vi "String_Parsing.vi"(7 "Search_Params":string[](array[string])=["x1", "y1", "z1", "x2", "y2", "z2"], 11 "Input":string) -> (3 "Positions":i32[](array[numeric]))   [LabVIEW 2016]
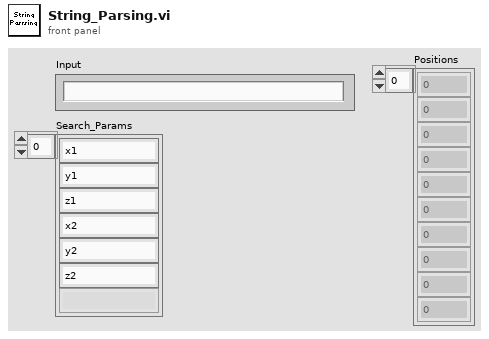
[diagram p1: front panel]
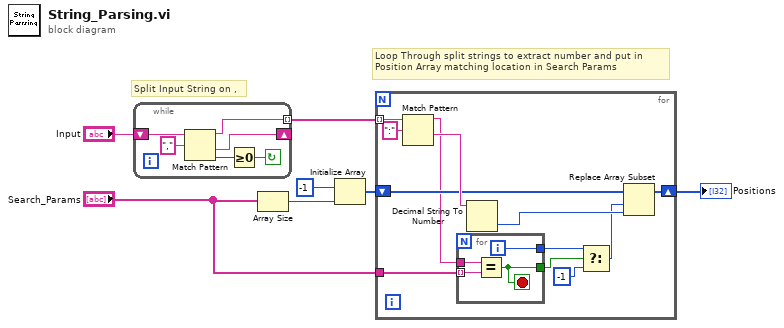
[diagram p0: block diagram]
diagram:
  # "Loop Through split strings to extract number and put in\nPosition Array matching location in Search Params"
  # "Split Input String on ,"
  n1 = while {
    shift-right: [w10] -> _
    shift-left: "Input" -> [w13]
    tunnel: [w11] -> w6 mode=indexing
    stop <- w8 continue-if-true
    n2 = Match Pattern(string=w13, regular expression=",") -> (before substring=w11:string, after substring=w10:string, offset past match=w9:i32)  [unwired: 1 in, 1 out]
    n3 = Greater Or Equal To 0?(x=w9) -> (x >= 0?=w8:bool)
  }
  n4 = Array Size(array="Search_Params") -> (size(s)=w1:i32)
  n5 = Initialize Array(-1 ("element"), w1) -> (w4:i32[])
  n6 = for {
    tunnel: w6 -> [w25] mode=indexing
    shift-right: [w21] -> w3
    shift-left: w4 -> [w22]
    tunnel: "Search_Params" -> [w18]
    n7 = Match Pattern(string=w25, regular expression=":") -> (before substring=w19:string, after substring=w23:string)  [unwired: 1 in, 2 out]
    n8 = for {
      tunnel: w19 -> [w29]
      tunnel: w18 -> [w28] mode=indexing
      tunnel: [w26] -> w17
      tunnel: [w27] -> w16
      i -> [w27]
      stop <- w26 stop-if-true
      n9 = Equal?(x=w29, y=w28) -> (x = y?=w26:bool)
    }
    n10 = Decimal String To Number(string=w23) -> (number=w20:i32)  [unwired: 2 in, 1 out]
    n11 = Select(t=w16, s=w17, f=-1) -> (s? t:f=w14:i32)
    n12 = Replace Array Subset(array=w22, new element=w20, index=w14) -> (w21:i32[])
  }
  "Positions" <- w3
